vi "GetTxRange.vi"(6 "Legacy (f)?":bool, 8 "error in (no error)":errorcluster) -> (0 "error out":errorcluster)   [LabVIEW 2011]
uses:
  HW Averaging.ctl
  PIM Parameters.ctl
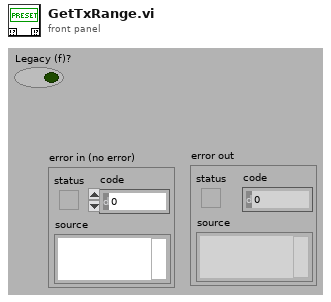
[diagram p1: front panel]
types:
  T1 = typedef "PIM Parameters.ctl" = enum16{"P11 (P1 Reflected)", "P12 (P2 Through)", "P21 (P1 Through)", "P22 (P2 Reflected)"}
  T2 = typedef "HW Averaging.ctl" = u16
  T3 = typedef "Test Set Definition.ctl" = cluster{"General":cluster{"ID":u32, "Model":string, "Dual Port?":bool, "Options":string, "Options":cluster{"E":bool, "K":bool, "H":bool, "W":bool, "F":bool}, "Cal File":path}, "Receiver":cluster{"Fstart, MHz":dbl, "Fstop MHz":dbl, "Fstep MHz":dbl, "IF, MHz":dbl}, "RX Band":cluster{"Fstart, MHz":dbl, "Fstop MHz":dbl}, "TX 1":cluster{"Fstart, MHz":dbl, "Fstop MHz":dbl, "Pmax, dBm":dbl, "Pstep, dB":dbl}, "TX 2":cluster{"Fstart, MHz":dbl, "Fstop MHz":dbl, "Pmax, dBm":dbl, "Pstep, dB":dbl}, "Low-side?":bool}
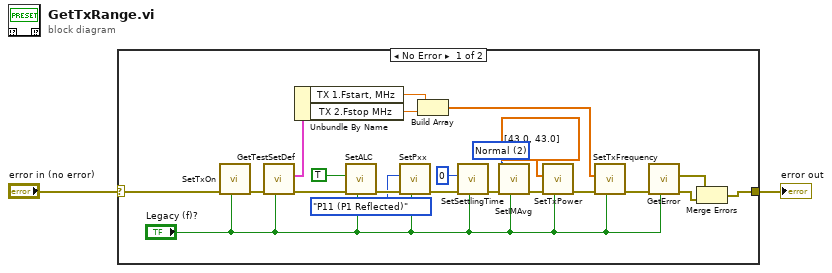
[diagram p0: block diagram]
diagram:
  n1 = case shown="No Error" "error in (no error)" {
    selector: "error in (no error)" -> [w6 w25]
    tunnel: [w4 w25] -> w2
    frame No Error {
      w14 = T2 2 items=["None", "Minimum", "Normal", "High", "Maximum"] ("SetIMAvg")
      n2 = call "SetTxOn.vi"("Legacy (f)?"="Legacy (f)?", "error in (no error)"=w6) -> ("error out"=w24:errorcluster)  [unwired: 8 in, 1 out]
      n3 = call "GetTestSetDef.vi"("Legacy (f)?"="Legacy (f)?", "error in (no error)"=w24) -> ("error out"=w19:errorcluster, "TestSetDef"=w23:T3)  [unwired: 8 in]
      n4 = Unbundle By Name(w23) -> ("TX 1.Fstart, MHz"=w22:dbl, "TX 2.Fstop MHz"=w21:dbl)
      n5 = call "SetALC.vi"("Legacy (f)?"="Legacy (f)?", "error in (no error)"=w19, "ALC"=TRUE) -> ("error out"=w18:errorcluster)  [unwired: 8 in]
      n6 = call "SetPxx.vi"("Legacy (f)?"="Legacy (f)?", "error in (no error)"=w18, "SetPxx"=PIM_Parameters."P11 (P1 Reflected)") -> ("error out"=w15:errorcluster)  [unwired: 8 in]
      n7 = Build Array(w22, w21) -> (w9:dbl[])
      n8 = call "SetSettlingTime.vi"("Legacy (f)?"="Legacy (f)?", "error in (no error)"=w15, "SettlingTime"=u32 0) -> ("error out"=w13:errorcluster)  [unwired: 8 in]
      n9 = call "SetIMAvg.vi"("Legacy (f)?"="Legacy (f)?", "error in (no error)"=w13, "SetIMAvg"=w14) -> ("error out"=w12:errorcluster)  [unwired: 8 in]
      n10 = call "SetTxPower.vi"("Legacy (f)?"="Legacy (f)?", "error in (no error)"=w12, "TxPower"=dbl[] [43.0, 43.0]) -> ("error out"=w10:errorcluster)  [unwired: 8 in]
      n11 = call "SetTxFrequency.vi"("Legacy (f)?"="Legacy (f)?", "error in (no error)"=w10, "TxFrequencies"=w9) -> ("error out"=w8:errorcluster)  [unwired: 8 in]
      n12 = call "GetError.vi"("Legacy (f)?"="Legacy (f)?", "error in (no error)"=w8) -> ("error out"=w5:errorcluster, "HW Error"=w3:errorcluster)  [unwired: 8 in]
      n13 = Merge Errors(w3, w5) -> (w4:errorcluster)
    }
    frame Error {
    }
  }
  "error out" <- w2
